vi "AnalysisTestCompile.vi"() -> ()   [LabVIEW 2013]
uses:
  <vilib>/Platform/TimedLoop/XDataNode/XDataNode.xnode
  <vilib>/Platform/TimedLoop/XDataNode/nitl_modes.ctl
  <vilib>/Platform/TimedLoop/XDataNode/XDNodeRunTimeDep.lvlib
  <vilib>/Platform/TimedLoop/XDataNode/wakeup.ctl
  <vilib>/Platform/TimedLoop/XDataNode/timing_clust.ctl
  <vilib>/rvi/DataTransferAndStorage/Container/XNode/niFpgaContainer.xnode
  <vilib>/rvi/FIFO/Fifo_Resource/nirvififoEmulationWrite.vi
panel:
  in  "Sector Threshold":u8
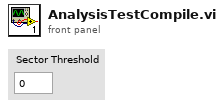
[diagram p1: front panel]
types:
  T1 = typedef "XDNodeRunTimeDep.lvlib/timing_clust.ctl" = cluster{"Expected End [f-1]":u64, "Actual End [f-1]":u64, "Finished Late? [f-1]":bool, "Expected End [i-1]":u64, "Actual End [i-1]":u64, "Finished Late? [i-1]":bool, "Expected Start [i]":u64, "Actual Start [i]":u64, "Expected Start [f]":u64, "Actual Start [f]":u64, "Source Name":string, "Structure Name":string, "Period":i64, "Deadline":i64, "Offset":i64, "Start":i64, "Priority":i32, "Timeout":i32, "Mode":T2, "Wakeup Reason":T3, "Error":errorcluster, "Source Type":string, "Secondary Source Type":string, "Global End Time":u64, "Global Start Time":u64, "Frame Duration":u64, "Iteration Duration":u64, "Assigned CPU":i32, "I/O Scan Engine Mode":u32}
  T2 = typedef "XDNodeRunTimeDep.lvlib/nitl_modes.ctl" = enum32{"No Change", "Process missed periods, maintain original phase", "Discard missed periods, maintain original phase", "Process missed periods, ignore original phase", "Discard missed periods, ignore original phase"}
  T3 = typedef "XDNodeRunTimeDep.lvlib/wakeup.ctl" = enum32{"Normal", "Aborted", "Asynchronous wakeup", "Timing source error", "Timed loop error", "Timeout"}
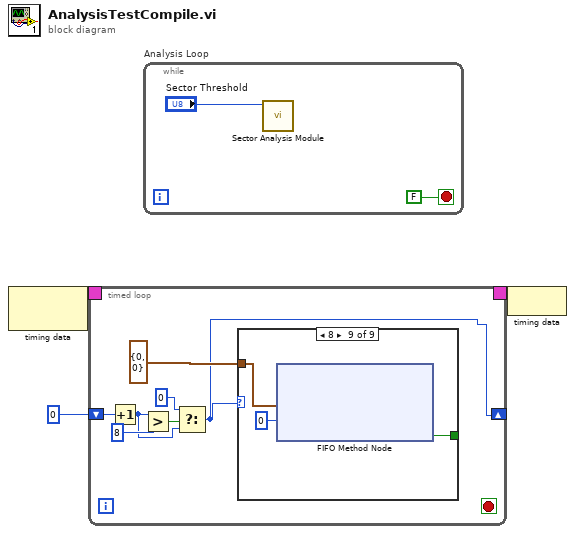
[diagram p0: block diagram]
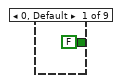
[diagram p2: hidden frame]
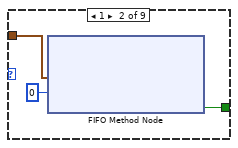
[diagram p3: hidden frame]
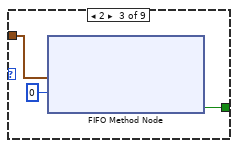
[diagram p4: hidden frame]
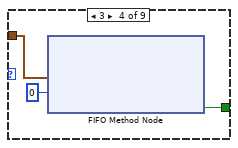
[diagram p5: hidden frame]
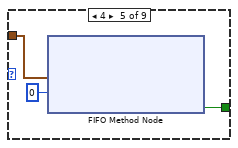
[diagram p6: hidden frame]
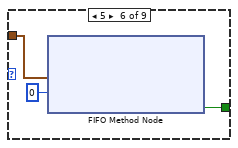
[diagram p7: hidden frame]
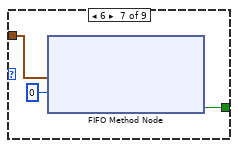
[diagram p8: hidden frame]
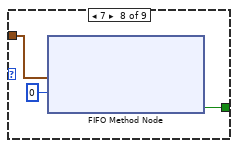
[diagram p9: hidden frame]
diagram:
  n1 = node-c288() -> (w3:T1)  [unwired: 1 in]
  n2 = timed-loop {
    timing: w3 -> [_]
    timing-out: [_] -> w2
    shift-right: [w4] -> _
    shift-left: u8 0 ("Current FIFO Check") -> [w9]
    stop <- _ stop-if-true
    n3 = Increment(x=w9) -> (x+1=w6:u8)
    n4 = Greater?(x=w6, y=u8 8) -> (0:w7:bool)
    n5 = Select(t=u8 0 ("y"), s=w7, f=w6) -> (s? t:f=w4:u8)
    n6 = case shown="8" w4 {
      tunnel: [FALSE ("Timed Out?") w13 w16 w19 w22 w25 w28 w31 w34] -> _
      tunnel: cluster{"Sector #":u8, "Pixel Value":u8} {"Sector #"=0, "Pixel Value"=0} ("Element") -> [_ w12 w15 w18 w21 w24 w27 w30 w33]
      frame 0, Default {
      }
      frame 1 {
        n7 = xnode ("FIFO Method Node")("Element"=w12, "Timeout"=0) -> ("Timed Out?"=w13:bool)  [unwired: 1 in, 1 out]
      }
      frame 2 {
        n8 = xnode ("FIFO Method Node")("Element"=w15, "Timeout"=0) -> ("Timed Out?"=w16:bool)  [unwired: 1 in, 1 out]
      }
      frame 3 {
        n9 = xnode ("FIFO Method Node")("Element"=w18, "Timeout"=0) -> ("Timed Out?"=w19:bool)  [unwired: 1 in, 1 out]
      }
      frame 4 {
        n10 = xnode ("FIFO Method Node")("Element"=w21, "Timeout"=0) -> ("Timed Out?"=w22:bool)  [unwired: 1 in, 1 out]
      }
      frame 5 {
        n11 = xnode ("FIFO Method Node")("Element"=w24, "Timeout"=0) -> ("Timed Out?"=w25:bool)  [unwired: 1 in, 1 out]
      }
      frame 6 {
        n12 = xnode ("FIFO Method Node")("Element"=w27, "Timeout"=0) -> ("Timed Out?"=w28:bool)  [unwired: 1 in, 1 out]
      }
      frame 7 {
        n13 = xnode ("FIFO Method Node")("Element"=w30, "Timeout"=0) -> ("Timed Out?"=w31:bool)  [unwired: 1 in, 1 out]
      }
      frame 8 {
        n14 = xnode ("FIFO Method Node")("Element"=w33, "Timeout"=0) -> ("Timed Out?"=w34:bool)  [unwired: 1 in, 1 out]
      }
    }
  }
  n15 = while "Analysis Loop" {
    stop <- FALSE stop-if-true
    n16 = call "Sector Analysis Module.vi"("Canceled?"="Sector Threshold") -> ()  [unwired: 6 in, 5 out]
  }
  n17 = node-c288(w2) -> ()
